vi "SpreadsheetStorage.vi"() -> ()   [LabVIEW 2014]
uses:
  <vilib>/Utility/file.llb/Write To Spreadsheet File (DBL).vi
panel:
  in  "Waveform Parameters":T1
  in  "Digitizing Parameters":T2
  out "XY Graph":cluster{"Time":dbl[], "Displacement":dbl[]}(graph)
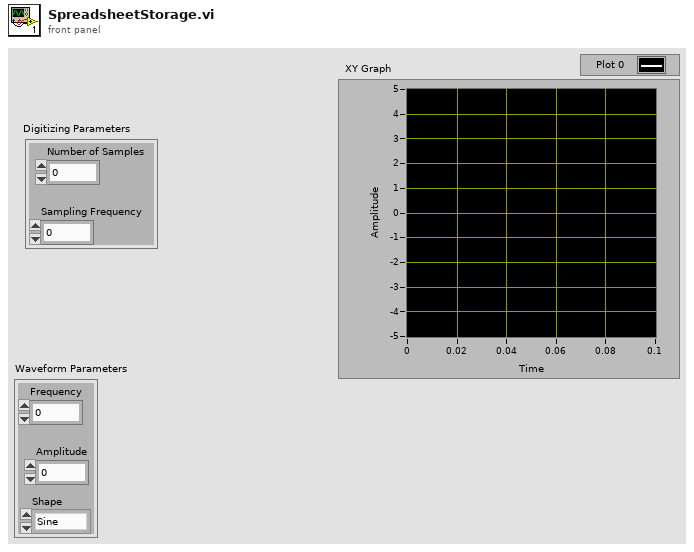
[diagram p1: front panel]
types:
  T1 = cluster{"Frequency":dbl, "Amplitude":dbl, "Shape":enum16{"Sine", "Cosine", "DC Level", "Square", "User-Defined"}}
  T2 = cluster{"Number of Samples":i32, "Sampling Frequency":dbl}
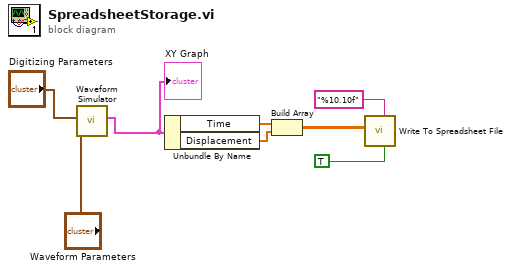
[diagram p0: block diagram]
diagram:
  n1 = call "Waveform Simulator.vi"("Waveform Parameters"="Waveform Parameters", "Digitizing Parameters"="Digitizing Parameters") -> ("Waveform Output"=w3:cluster{"Time":dbl[], "Displacement":dbl[]})  [unwired: 9 in]
  "XY Graph" <- w3
  n2 = Unbundle By Name(w3) -> ("Time"=w8:dbl[], "Displacement"=w7:dbl[])
  n3 = Build Array(w8, w7) -> (w6:dbl[][])
  n4 = call-poly <vilib>:"Write To Spreadsheet File.vi"("transpose? (no:F)"=TRUE, "format (%.3f)"="%10.10f", "2D data"=w6) -> ()  [unwired: 5 in, 1 out]
